vi "Clear Data.vi"(8 "error in (no error)":errorcluster, 10 "Clear Data Type (0:All)":u16(ring) items=["All", "Target Volume", "Target Time", "Infused & Withdrawn Volume", "Infused & Withdrawn Time"], 11 "VISA resource name":refnum<visa-resource-name>) -> (0 "error out":errorcluster, 3 "VISA resource name out":refnum<visa-resource-name>)   [LabVIEW 2016]
doc: "Clears Target Volume, Target Time, Infused & Withdrawn Volume and Time or All."
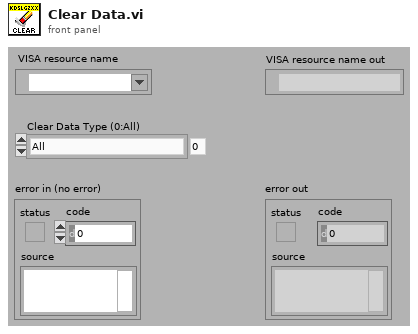
[diagram p1: front panel]
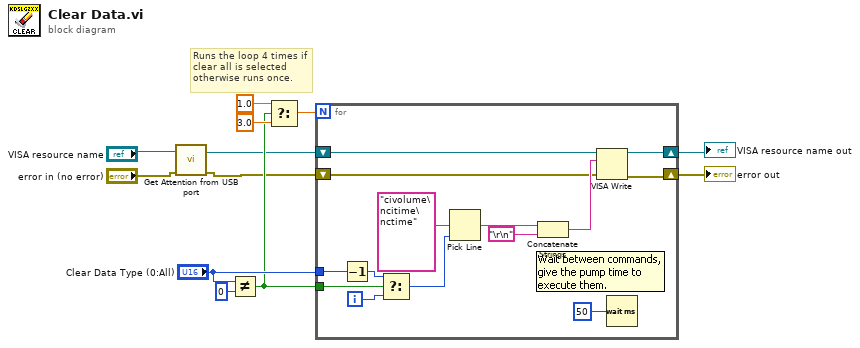
[diagram p0: block diagram]
diagram:
  # "Runs the loop 4 times if clear all is selected otherwise runs once."
  n1 = call "Get Attention from USB port.vi"("error in (no error)"="error in (no error)", "VISA resource name"="VISA resource name") -> ("error out"=w3:errorcluster, "VISA resource name out"=w4:refnum<visa-resource-name>)  [unwired: 8 in]
  n2 = Not Equal?(x="Clear Data Type (0:All)", y=u16 0) -> (x != y?=w5:bool)
  n3 = Select(t=1.0, s=w5, f=3.0) -> (s? t:f=w11:dbl)
  n4 = for {
    N: w11 -> [_]
    tunnel: w5 -> [w25]
    shift-right: [w24] -> w8
    shift-left: w4 -> [w15]
    shift-right: [w23] -> w7
    shift-left: w3 -> [w14]
    tunnel: "Clear Data Type (0:All)" -> [w18]
    i -> [w16]
    n5 = Decrement(x=w18) -> (x-1=w17:u16)
    n6 = Select(t=w17, s=w25, f=w16) -> (s? t:f=w22:i32)
    n7 = Pick Line(multi-line string="civolume\ncitime\nctime", line index=w22) -> (output string=w21:string)  [unwired: 1 in]
    n8 = Concatenate Strings(w21, "\r\n") -> (w19:string)
    n9 = VISA Write(VISA resource name=w15, write buffer=w19, error in (no error)=w14) -> (VISA resource name out=w24:refnum<visa-resource-name>, error out=w23:errorcluster)  [unwired: 1 out]
    n10 = Wait (ms)(milliseconds to wait=u32 50) -> ()  [unwired: 1 out]
  }
  "VISA resource name out" <- w8
  "error out" <- w7
